vi "Gather data from device.vi"(2 "error in (no error)":errorcluster, 3 "Front Panel Object References":T1) -> (0 "error out":errorcluster)   [LabVIEW 2020]
uses:
  Typedefs/Front Panel Object References.ctl
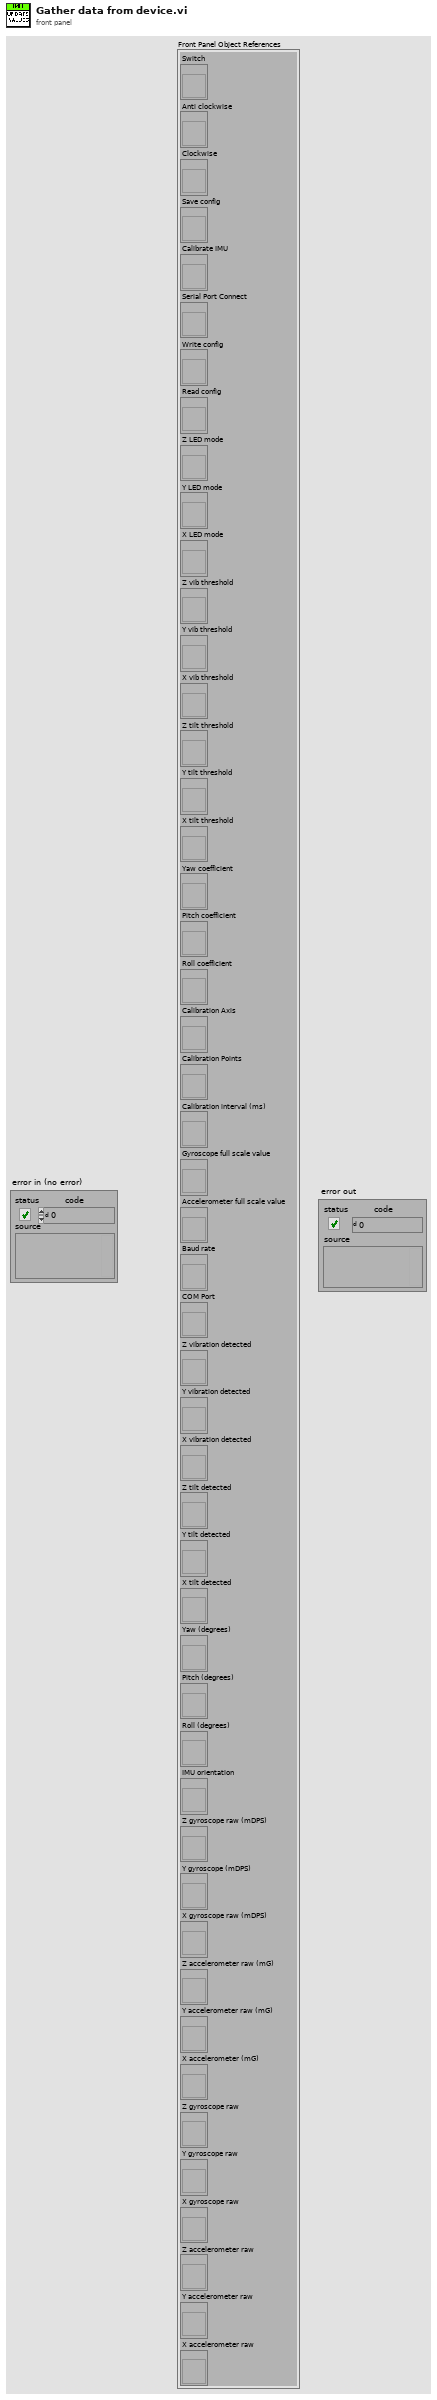
[diagram p1: front panel]
types:
  T1 = typedef "Front Panel Object References.ctl" = cluster{"Switch":refnum<vi>, "Anti clockwise":refnum<vi>, "Clockwise":refnum<vi>, "Save config":refnum<vi>, "Calibrate IMU":refnum<vi>, "Serial Port Connect":refnum<vi>, "Write config":refnum<vi>, "Read config":refnum<vi>, "Z LED mode":refnum<vi>, "Y LED mode":refnum<vi>, "X LED mode":refnum<vi>, "Z vib threshold":refnum<vi>, "Y vib threshold":refnum<vi>, "X vib threshold":refnum<vi>, "Z tilt threshold":refnum<vi>, "Y tilt threshold":refnum<vi>, "X tilt threshold":refnum<vi>, "Yaw coefficient":refnum<vi>, "Pitch coefficient":refnum<vi>, "Roll coefficient":refnum<vi>, "Calibration Axis":refnum<vi>, "Calibration Points":refnum<vi>, "Calibration interval (ms)":refnum<vi>, "Gyroscope full scale value":refnum<vi>, "Accelerometer full scale value":refnum<vi>, "Baud rate":refnum<vi>, "COM Port":refnum<vi>, "Z vibration detected":refnum<vi>, "Y vibration detected":refnum<vi>, "X vibration detected":refnum<vi>, "Z tilt detected":refnum<vi>, "Y tilt detected":refnum<vi>, "X tilt detected":refnum<vi>, "Yaw (degrees)":refnum<vi>, "Pitch (degrees)":refnum<vi>, "Roll (degrees)":refnum<vi>, "IMU orientation":refnum<vi>, "Z gyroscope raw (mDPS)":refnum<vi>, "Y gyroscope (mDPS)":refnum<vi>, "X gyroscope raw (mDPS)":refnum<vi>, "Z accelerometer raw (mG)":refnum<vi>, "Y accelerometer raw (mG)":refnum<vi>, "X accelerometer (mG)":refnum<vi>, "Z gyroscope raw":refnum<vi>, "Y gyroscope raw":refnum<vi>, "X gyroscope raw":refnum<vi>, "Z accelerometer raw":refnum<vi>, "Y accelerometer raw":refnum<vi>, "X accelerometer raw":refnum<vi>}
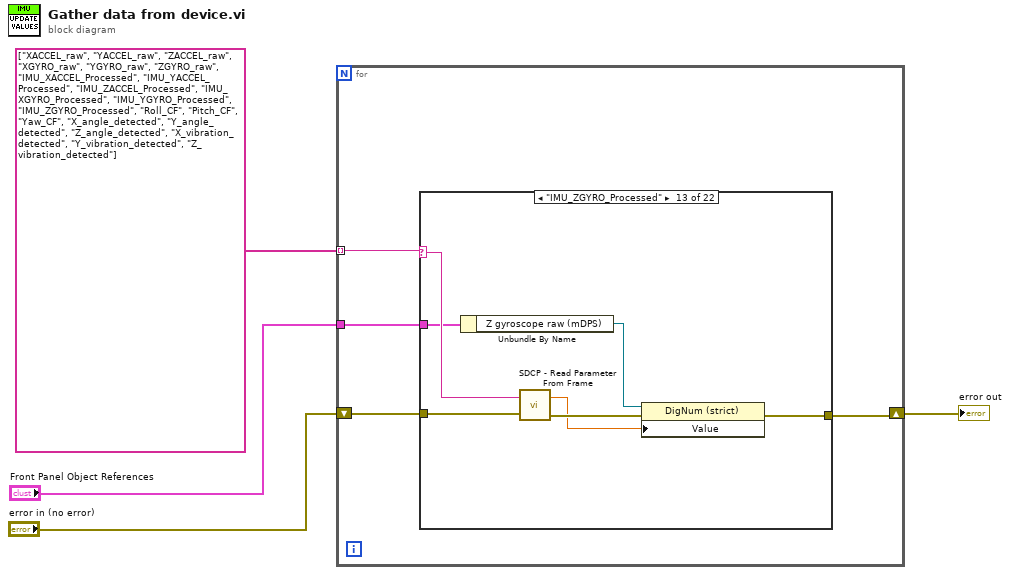
[diagram p0: block diagram]
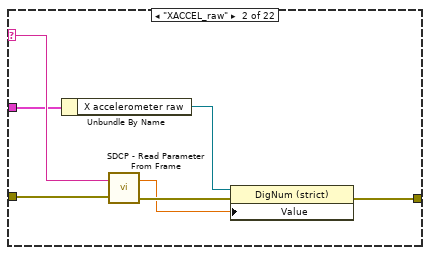
[diagram p3: hidden frame]
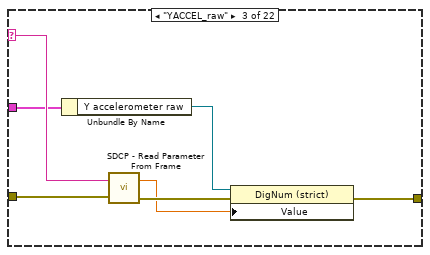
[diagram p4: hidden frame]
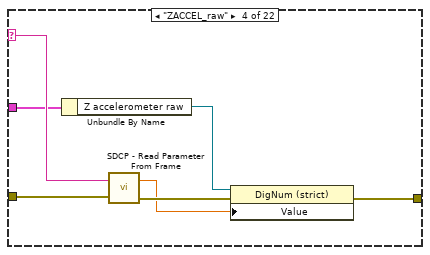
[diagram p5: hidden frame]
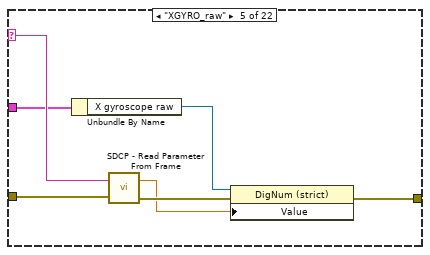
[diagram p6: hidden frame]
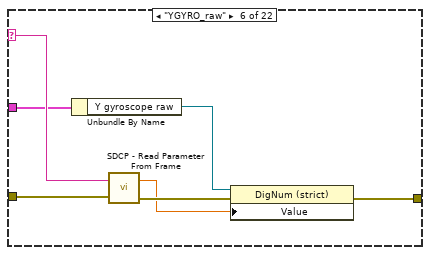
[diagram p7: hidden frame]
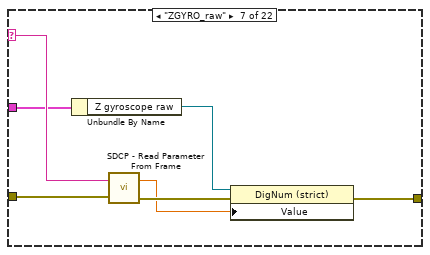
[diagram p8: hidden frame]
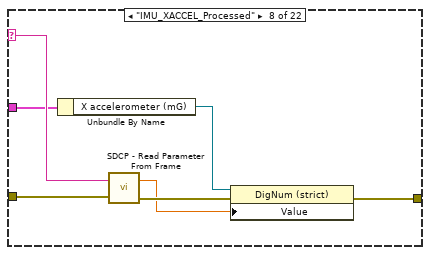
[diagram p9: hidden frame]
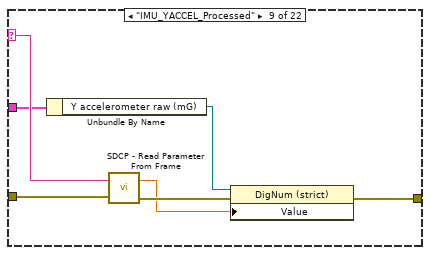
[diagram p10: hidden frame]
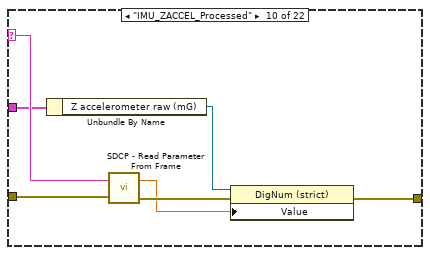
[diagram p11: hidden frame]
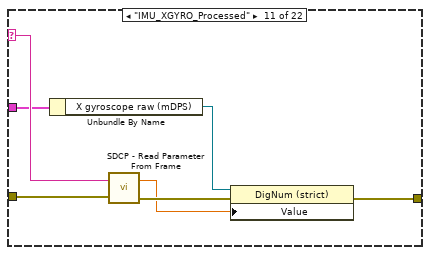
[diagram p12: hidden frame]
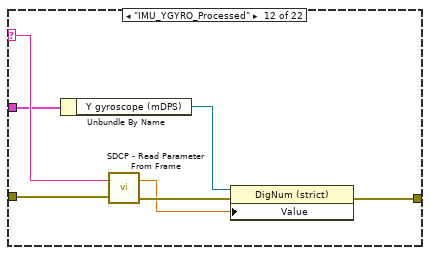
[diagram p13: hidden frame]
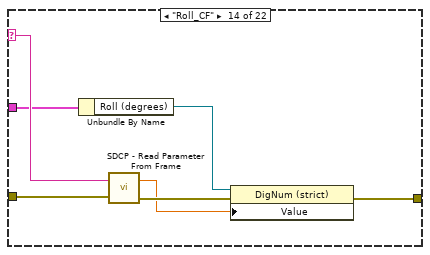
[diagram p14: hidden frame]
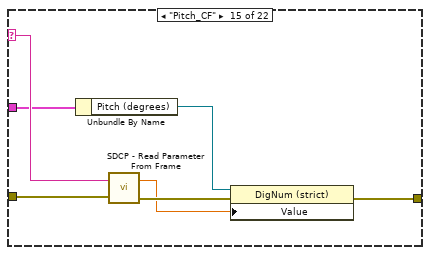
[diagram p15: hidden frame]
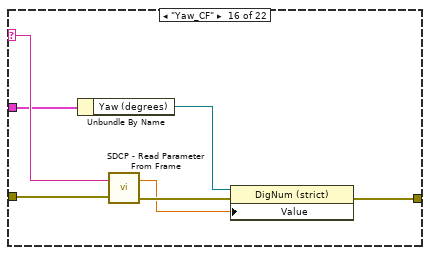
[diagram p16: hidden frame]
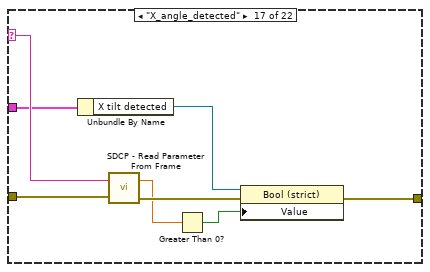
[diagram p17: hidden frame]
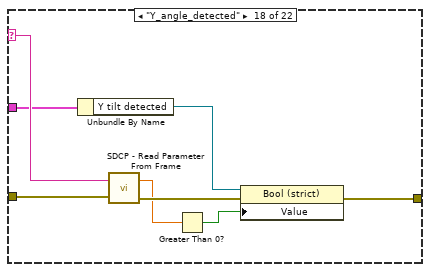
[diagram p18: hidden frame]
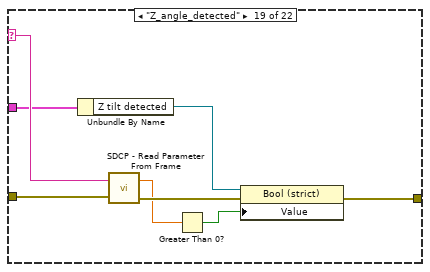
[diagram p19: hidden frame]
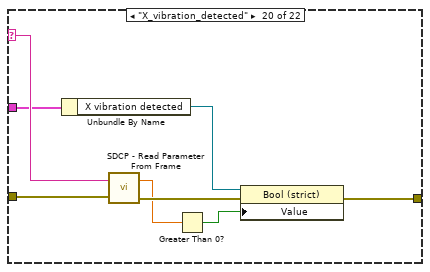
[diagram p20: hidden frame]
diagram:
  n1 = for {
    tunnel: string[] ["XACCEL_raw", "YACCEL_raw", "ZACCEL_raw", "XGYRO_raw", "YGYRO_raw", "ZGYRO_raw", "IMU_XACCEL_Processed", "IMU_YACCEL_Processed", "IMU_ZACCEL_Processed", "IMU_XGYRO_Processed", "IMU_YGYRO_Processed", "IMU_ZGYRO_Processed", "Roll_CF", "Pitch_CF", "Yaw_CF", "X_angle_detected", "Y_angle_detected", "Z_angle_detected", "X_vibration_detected", "Y_vibration_detected", "Z_vibration_detected"] -> [w8] mode=indexing
    tunnel: "Front Panel Object References" -> [w6]
    shift-right: [w5] -> w1
    shift-left: "error in (no error)" -> [w7]
    n2 = case shown="\"IMU_ZGYRO_Processed\"" w8 {
      selector: w8 -> [_ w15 w22 w29 w36 w43 w50 w57 w64 w71 w78 w85 w92 w99 w106 w113 w121 w129 w137 w145 w153 w161]
      tunnel: w7 -> [w9 w16 w23 w30 w37 w44 w51 w58 w65 w72 w79 w86 w93 w100 w107 w114 w122 w130 w138 w146 w154 w162]
      tunnel: w6 -> [_ w14 w21 w28 w35 w42 w49 w56 w63 w70 w77 w84 w91 w98 w105 w112 w120 w128 w136 w144 w152 w160]
      tunnel: [w9 w10 w17 w24 w31 w38 w45 w52 w59 w66 w73 w80 w87 w94 w101 w108 w117 w125 w133 w141 w149 w157] -> w5
      frame Default {
      }
      frame "XACCEL_raw" {
        n3 = Unbundle By Name(w14) -> ("X accelerometer raw"=w12:refnum<vi>)
        n4 = call "SDCP - Read Parameter From Frame.vi"("error in (no error)"=w16, "Parameter"=w15) -> ("error out"=w13:errorcluster, "Value"=w11:dbl)
        n5 = property class="DigNum (strict)"(reference=w12, error in=w13, "Value"=w11) -> (error out=w10:errorcluster)  [unwired: 1 out]
      }
      frame "YACCEL_raw" {
        n6 = Unbundle By Name(w21) -> ("Y accelerometer raw"=w19:refnum<vi>)
        n7 = call "SDCP - Read Parameter From Frame.vi"("error in (no error)"=w23, "Parameter"=w22) -> ("error out"=w20:errorcluster, "Value"=w18:dbl)
        n8 = property class="DigNum (strict)"(reference=w19, error in=w20, "Value"=w18) -> (error out=w17:errorcluster)  [unwired: 1 out]
      }
      frame "ZACCEL_raw" {
        n9 = Unbundle By Name(w28) -> ("Z accelerometer raw"=w26:refnum<vi>)
        n10 = call "SDCP - Read Parameter From Frame.vi"("error in (no error)"=w30, "Parameter"=w29) -> ("error out"=w27:errorcluster, "Value"=w25:dbl)
        n11 = property class="DigNum (strict)"(reference=w26, error in=w27, "Value"=w25) -> (error out=w24:errorcluster)  [unwired: 1 out]
      }
      frame "XGYRO_raw" {
        n12 = Unbundle By Name(w35) -> ("X gyroscope raw"=w33:refnum<vi>)
        n13 = call "SDCP - Read Parameter From Frame.vi"("error in (no error)"=w37, "Parameter"=w36) -> ("error out"=w34:errorcluster, "Value"=w32:dbl)
        n14 = property class="DigNum (strict)"(reference=w33, error in=w34, "Value"=w32) -> (error out=w31:errorcluster)  [unwired: 1 out]
      }
      frame "YGYRO_raw" {
        n15 = Unbundle By Name(w42) -> ("Y gyroscope raw"=w40:refnum<vi>)
        n16 = call "SDCP - Read Parameter From Frame.vi"("error in (no error)"=w44, "Parameter"=w43) -> ("error out"=w41:errorcluster, "Value"=w39:dbl)
        n17 = property class="DigNum (strict)"(reference=w40, error in=w41, "Value"=w39) -> (error out=w38:errorcluster)  [unwired: 1 out]
      }
      frame "ZGYRO_raw" {
        n18 = Unbundle By Name(w49) -> ("Z gyroscope raw"=w47:refnum<vi>)
        n19 = call "SDCP - Read Parameter From Frame.vi"("error in (no error)"=w51, "Parameter"=w50) -> ("error out"=w48:errorcluster, "Value"=w46:dbl)
        n20 = property class="DigNum (strict)"(reference=w47, error in=w48, "Value"=w46) -> (error out=w45:errorcluster)  [unwired: 1 out]
      }
      frame "IMU_XACCEL_Processed" {
        n21 = Unbundle By Name(w56) -> ("X accelerometer (mG)"=w54:refnum<vi>)
        n22 = call "SDCP - Read Parameter From Frame.vi"("error in (no error)"=w58, "Parameter"=w57) -> ("error out"=w55:errorcluster, "Value"=w53:dbl)
        n23 = property class="DigNum (strict)"(reference=w54, error in=w55, "Value"=w53) -> (error out=w52:errorcluster)  [unwired: 1 out]
      }
      frame "IMU_YACCEL_Processed" {
        n24 = Unbundle By Name(w63) -> ("Y accelerometer raw (mG)"=w61:refnum<vi>)
        n25 = call "SDCP - Read Parameter From Frame.vi"("error in (no error)"=w65, "Parameter"=w64) -> ("error out"=w62:errorcluster, "Value"=w60:dbl)
        n26 = property class="DigNum (strict)"(reference=w61, error in=w62, "Value"=w60) -> (error out=w59:errorcluster)  [unwired: 1 out]
      }
      frame "IMU_ZACCEL_Processed" {
        n27 = Unbundle By Name(w70) -> ("Z accelerometer raw (mG)"=w68:refnum<vi>)
        n28 = call "SDCP - Read Parameter From Frame.vi"("error in (no error)"=w72, "Parameter"=w71) -> ("error out"=w69:errorcluster, "Value"=w67:dbl)
        n29 = property class="DigNum (strict)"(reference=w68, error in=w69, "Value"=w67) -> (error out=w66:errorcluster)  [unwired: 1 out]
      }
      frame "IMU_XGYRO_Processed" {
        n30 = Unbundle By Name(w77) -> ("X gyroscope raw (mDPS)"=w75:refnum<vi>)
        n31 = call "SDCP - Read Parameter From Frame.vi"("error in (no error)"=w79, "Parameter"=w78) -> ("error out"=w76:errorcluster, "Value"=w74:dbl)
        n32 = property class="DigNum (strict)"(reference=w75, error in=w76, "Value"=w74) -> (error out=w73:errorcluster)  [unwired: 1 out]
      }
      frame "IMU_YGYRO_Processed" {
        n33 = Unbundle By Name(w84) -> ("Y gyroscope (mDPS)"=w82:refnum<vi>)
        n34 = call "SDCP - Read Parameter From Frame.vi"("error in (no error)"=w86, "Parameter"=w85) -> ("error out"=w83:errorcluster, "Value"=w81:dbl)
        n35 = property class="DigNum (strict)"(reference=w82, error in=w83, "Value"=w81) -> (error out=w80:errorcluster)  [unwired: 1 out]
      }
      frame "IMU_ZGYRO_Processed" {
        n36 = Unbundle By Name(w91) -> ("Z gyroscope raw (mDPS)"=w89:refnum<vi>)
        n37 = call "SDCP - Read Parameter From Frame.vi"("error in (no error)"=w93, "Parameter"=w92) -> ("error out"=w90:errorcluster, "Value"=w88:dbl)
        n38 = property class="DigNum (strict)"(reference=w89, error in=w90, "Value"=w88) -> (error out=w87:errorcluster)  [unwired: 1 out]
      }
      frame "Roll_CF" {
        n39 = Unbundle By Name(w98) -> ("Roll (degrees)"=w96:refnum<vi>)
        n40 = call "SDCP - Read Parameter From Frame.vi"("error in (no error)"=w100, "Parameter"=w99) -> ("error out"=w97:errorcluster, "Value"=w95:dbl)
        n41 = property class="DigNum (strict)"(reference=w96, error in=w97, "Value"=w95) -> (error out=w94:errorcluster)  [unwired: 1 out]
      }
      frame "Pitch_CF" {
        n42 = Unbundle By Name(w105) -> ("Pitch (degrees)"=w103:refnum<vi>)
        n43 = call "SDCP - Read Parameter From Frame.vi"("error in (no error)"=w107, "Parameter"=w106) -> ("error out"=w104:errorcluster, "Value"=w102:dbl)
        n44 = property class="DigNum (strict)"(reference=w103, error in=w104, "Value"=w102) -> (error out=w101:errorcluster)  [unwired: 1 out]
      }
      frame "Yaw_CF" {
        n45 = Unbundle By Name(w112) -> ("Yaw (degrees)"=w110:refnum<vi>)
        n46 = call "SDCP - Read Parameter From Frame.vi"("error in (no error)"=w114, "Parameter"=w113) -> ("error out"=w111:errorcluster, "Value"=w109:dbl)
        n47 = property class="DigNum (strict)"(reference=w110, error in=w111, "Value"=w109) -> (error out=w108:errorcluster)  [unwired: 1 out]
      }
      frame "X_angle_detected" {
        n48 = Unbundle By Name(w120) -> ("X tilt detected"=w118:refnum<vi>)
        n49 = call "SDCP - Read Parameter From Frame.vi"("error in (no error)"=w122, "Parameter"=w121) -> ("error out"=w119:errorcluster, "Value"=w116:dbl)
        n50 = Greater Than 0?(x=w116) -> (x > 0?=w115:bool)
        n51 = property class="Bool (strict)"(reference=w118, error in=w119, "Value"=w115) -> (error out=w117:errorcluster)  [unwired: 1 out]
      }
      frame "Y_angle_detected" {
        n52 = Unbundle By Name(w128) -> ("Y tilt detected"=w126:refnum<vi>)
        n53 = call "SDCP - Read Parameter From Frame.vi"("error in (no error)"=w130, "Parameter"=w129) -> ("error out"=w127:errorcluster, "Value"=w124:dbl)
        n54 = Greater Than 0?(x=w124) -> (x > 0?=w123:bool)
        n55 = property class="Bool (strict)"(reference=w126, error in=w127, "Value"=w123) -> (error out=w125:errorcluster)  [unwired: 1 out]
      }
      frame "Z_angle_detected" {
        n56 = Unbundle By Name(w136) -> ("Z tilt detected"=w134:refnum<vi>)
        n57 = call "SDCP - Read Parameter From Frame.vi"("error in (no error)"=w138, "Parameter"=w137) -> ("error out"=w135:errorcluster, "Value"=w132:dbl)
        n58 = Greater Than 0?(x=w132) -> (x > 0?=w131:bool)
        n59 = property class="Bool (strict)"(reference=w134, error in=w135, "Value"=w131) -> (error out=w133:errorcluster)  [unwired: 1 out]
      }
      frame "X_vibration_detected" {
        n60 = Unbundle By Name(w144) -> ("X vibration detected"=w142:refnum<vi>)
        n61 = call "SDCP - Read Parameter From Frame.vi"("error in (no error)"=w146, "Parameter"=w145) -> ("error out"=w143:errorcluster, "Value"=w140:dbl)
        n62 = Greater Than 0?(x=w140) -> (x > 0?=w139:bool)
        n63 = property class="Bool (strict)"(reference=w142, error in=w143, "Value"=w139) -> (error out=w141:errorcluster)  [unwired: 1 out]
      }
      frame "Y_vibration_detected" {
        n64 = Unbundle By Name(w152) -> ("Y vibration detected"=w150:refnum<vi>)
        n65 = call "SDCP - Read Parameter From Frame.vi"("error in (no error)"=w154, "Parameter"=w153) -> ("error out"=w151:errorcluster, "Value"=w148:dbl)
        n66 = Greater Than 0?(x=w148) -> (x > 0?=w147:bool)
        n67 = property class="Bool (strict)"(reference=w150, error in=w151, "Value"=w147) -> (error out=w149:errorcluster)  [unwired: 1 out]
      }
      frame "Z_vibration_detected" {
        n68 = Unbundle By Name(w160) -> ("Z vibration detected"=w158:refnum<vi>)
        n69 = call "SDCP - Read Parameter From Frame.vi"("error in (no error)"=w162, "Parameter"=w161) -> ("error out"=w159:errorcluster, "Value"=w156:dbl)
        n70 = Greater Than 0?(x=w156) -> (x > 0?=w155:bool)
        n71 = property class="Bool (strict)"(reference=w158, error in=w159, "Value"=w155) -> (error out=w157:errorcluster)  [unwired: 1 out]
      }
    }
  }
  "error out" <- w1
